vi "ring_buoy_ring.vi"(8 "error in (no error)":errorcluster, 11 "Image":T1) -> (0 "error out":errorcluster, 2 "circular particles":dbl[][](array[numeric]), 3 "Image Dst Out":T1)   [LabVIEW 2009]
uses:
  <vilib>/vision/Image Controls.llb/IMAQ Image.ctl
  <vilib>/vision/NI_Vision_Development_Module.lvlib
panel:
  out "size(s)":i32[](array[numeric])
  out "Particle Measurements (Pixels)":dbl[][](array[numeric]) format="%.2f"
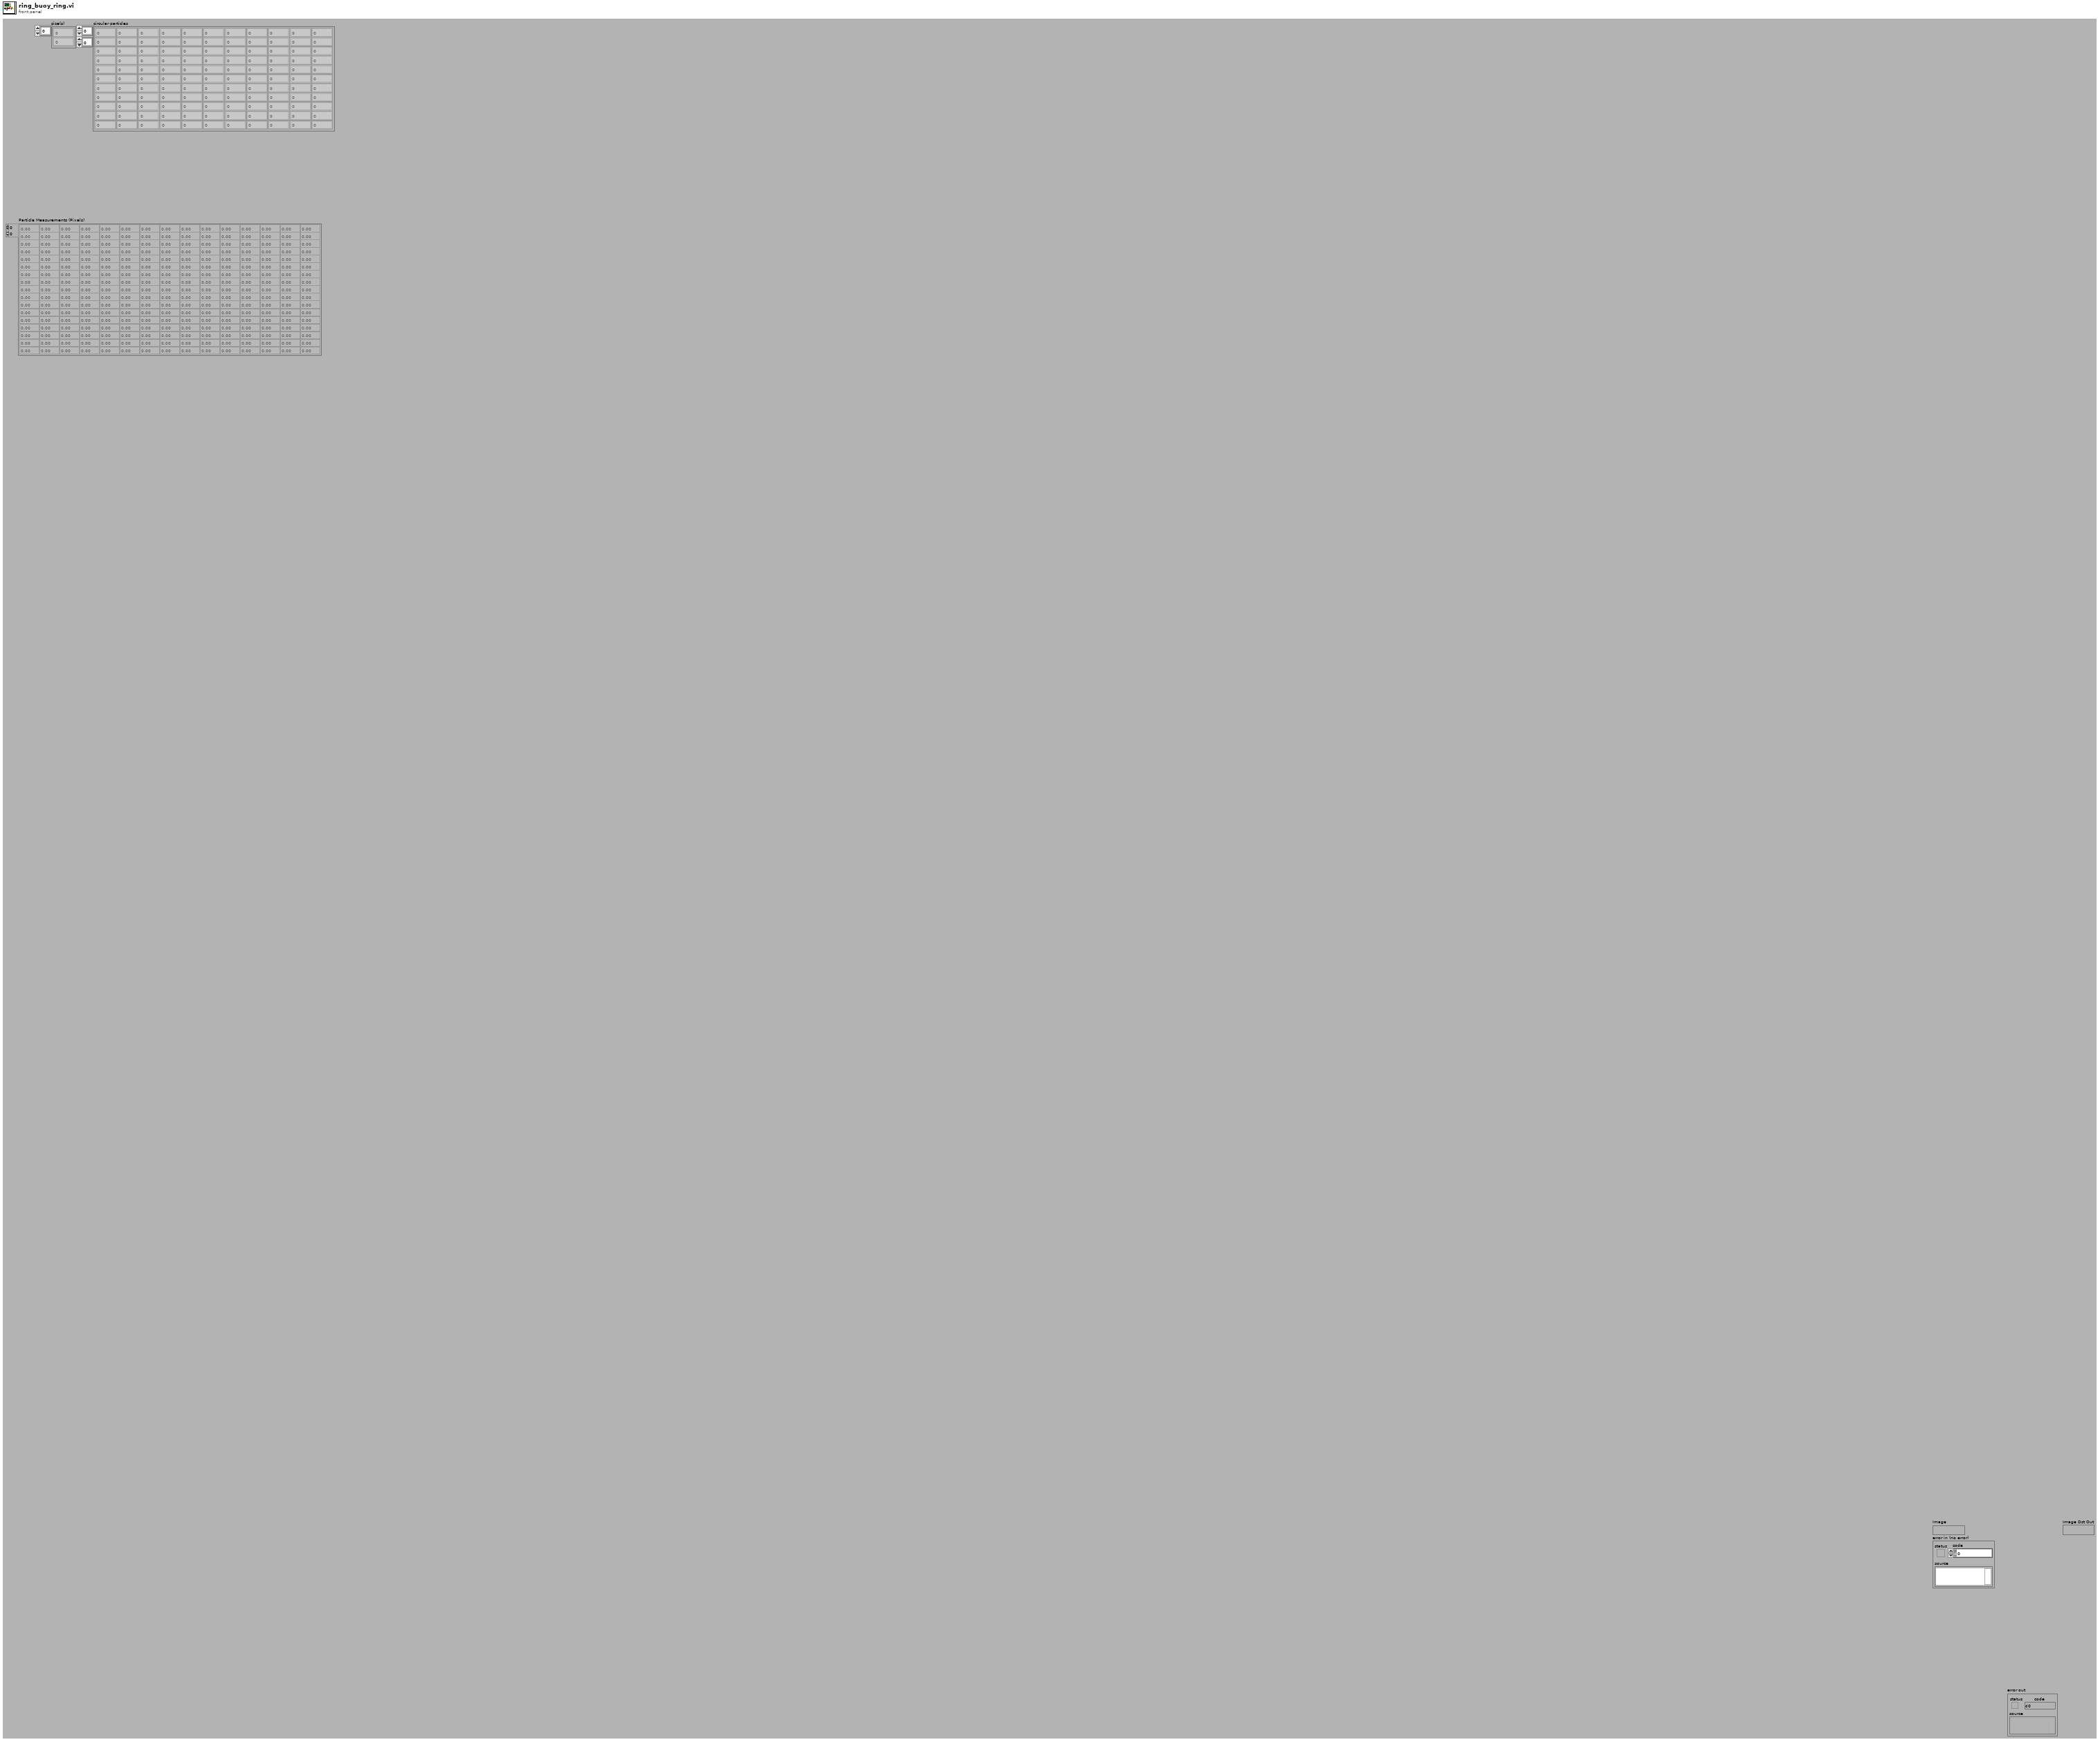
[diagram p1: front panel]
types:
  T1 = typedef "IMAQ Image.ctl" = refnum<image>
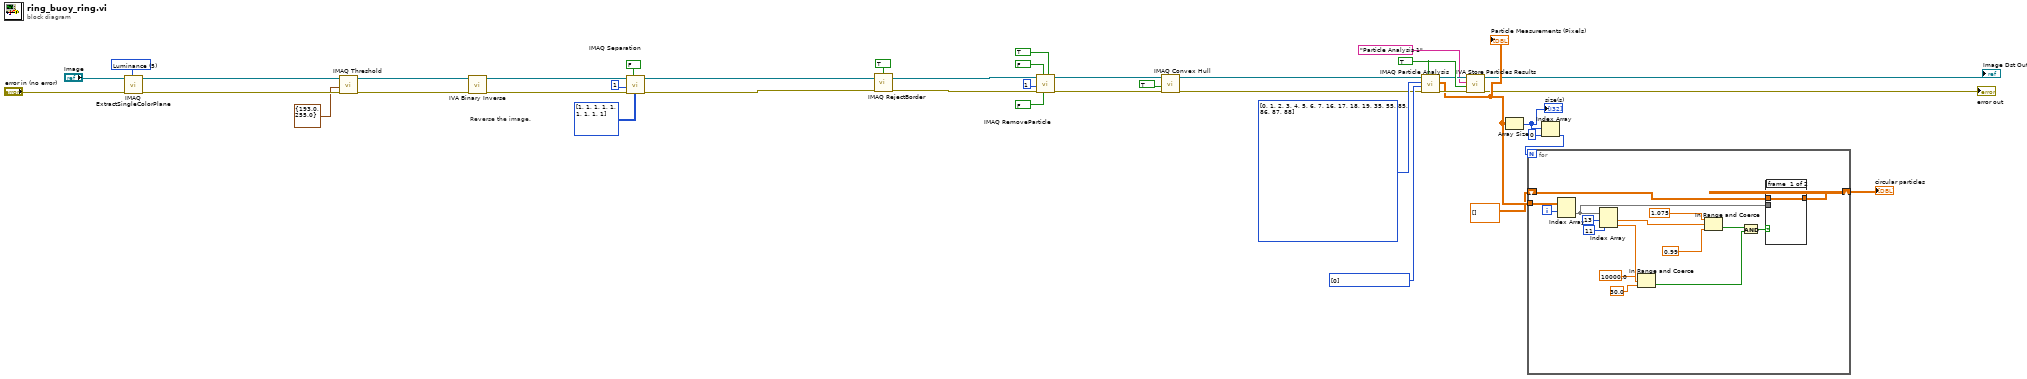
[diagram p0: block diagram]
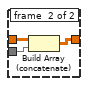
[diagram p2: hidden frame]
diagram:
  w16 = i32[] [0] items=["Center of Mass X", "Center of Mass Y", "First Pixel X", "First Pixel Y", "Bounding Rect Left", "Bounding Rect Top", "Bounding Rect Right", "Bounding Rect Bottom", "Max Feret Diameter Start X", "Max Feret Diameter Start Y", "Max Feret Diameter End X", "Max Feret Diameter End Y", "Max Horiz. Segment Length Left", "Max Horiz. Segment Length Right", "Max Horiz. Segment Length Row", "-", "Bounding Rect Width", "Bounding Rect Height", "Bounding Rect Diagonal", "Perimeter", "Convex Hull Perimeter", "Holes' Perimeter", "Max Feret Diameter", "Equivalent Ellipse Major Axis", "Equivalent Ellipse Minor Axis", "Equivalent Ellipse Minor Axis (Feret)", "Equivalent Rect Long Side", "Equivalent Rect Short Side", "Equivalent Rect Diagonal", "Equivalent Rect Short Side (Feret)", "Average Horiz. Segment Length", "Average Vert. Segment Length", "Hydraulic Radius", "Waddel Disk Diameter", "-", "Area", "Holes' Area", "Particle & Holes' Area", "Convex Hull Area", "Image Area", "-", "Number of Holes", "Number of Horiz. Segments", "Number of Vert. Segments", "-", "Orientation", "Max Feret Diameter Orientation", "-", "% Area/Image Area", "% Area/(Particle & Holes' Area)", "Ratio of Equivalent Ellipse Axes", "Ratio of Equivalent Rect Sides", "-", "Elongation Factor", "Compactness Factor", "Heywood Circularity Factor", "Type Factor", "-", "Sum X", "Sum Y", "Sum XX", "Sum XY", "Sum YY", "Sum XXX", "Sum XXY", "Sum XYY", "Sum YYY", "-", "Moment of Inertia XX", "Moment of Inertia XY", "Moment of Inertia YY", "Moment of Inertia XXX", "Moment of Inertia XXY", "Moment of Inertia XYY", "Moment of Inertia YYY", "Norm. Moment of Inertia XX", "Norm. Moment of Inertia XY", "Norm. Moment of Inertia YY", "Norm. Moment of Inertia XXX", "Norm. Moment of Inertia XXY", "Norm. Moment of Inertia XYY", "Norm. Moment of Inertia YYY", "Hu Moment 1", "Hu Moment 2", "Hu Moment 3", "Hu Moment 4", "Hu Moment 5", "Hu Moment 6", "Hu Moment 7"] ("Real-World Measurements")
  w11 = i32[] [0, 1, 2, 3, 4, 5, 6, 7, 16, 17, 18, 19, 35, 55, 85, 86, 87, 88] items=["Center of Mass X", "Center of Mass Y", "First Pixel X", "First Pixel Y", "Bounding Rect Left", "Bounding Rect Top", "Bounding Rect Right", "Bounding Rect Bottom", "Max Feret Diameter Start X", "Max Feret Diameter Start Y", "Max Feret Diameter End X", "Max Feret Diameter End Y", "Max Horiz. Segment Length Left", "Max Horiz. Segment Length Right", "Max Horiz. Segment Length Row", "-", "Bounding Rect Width", "Bounding Rect Height", "Bounding Rect Diagonal", "Perimeter", "Convex Hull Perimeter", "Holes' Perimeter", "Max Feret Diameter", "Equivalent Ellipse Major Axis", "Equivalent Ellipse Minor Axis", "Equivalent Ellipse Minor Axis (Feret)", "Equivalent Rect Long Side", "Equivalent Rect Short Side", "Equivalent Rect Diagonal", "Equivalent Rect Short Side (Feret)", "Average Horiz. Segment Length", "Average Vert. Segment Length", "Hydraulic Radius", "Waddel Disk Diameter", "-", "Area", "Holes' Area", "Particle & Holes' Area", "Convex Hull Area", "Image Area", "-", "Number of Holes", "Number of Horiz. Segments", "Number of Vert. Segments", "-", "Orientation", "Max Feret Diameter Orientation", "-", "% Area/Image Area", "% Area/(Particle & Holes' Area)", "Ratio of Equivalent Ellipse Axes", "Ratio of Equivalent Rect Sides", "-", "Elongation Factor", "Compactness Factor", "Heywood Circularity Factor", "Type Factor", "-", "Sum X", "Sum Y", "Sum XX", "Sum XY", "Sum YY", "Sum XXX", "Sum XXY", "Sum XYY", "Sum YYY", "-", "Moment of Inertia XX", "Moment of Inertia XY", "Moment of Inertia YY", "Moment of Inertia XXX", "Moment of Inertia XXY", "Moment of Inertia XYY", "Moment of Inertia YYY", "Norm. Moment of Inertia XX", "Norm. Moment of Inertia XY", "Norm. Moment of Inertia YY", "Norm. Moment of Inertia XXX", "Norm. Moment of Inertia XXY", "Norm. Moment of Inertia XYY", "Norm. Moment of Inertia YYY", "Hu Moment 1", "Hu Moment 2", "Hu Moment 3", "Hu Moment 4", "Hu Moment 5", "Hu Moment 6", "Hu Moment 7"] ("Pixel Measurements")
  w15 = TRUE ("Connectivity 4/8 (8)")
  w41 = 5 items=["Red", "Green", "Blue", "Hue", "Saturation", "Luminance", "Value", "Intensity"] ("Color Plane")
  # "Reverse the image."
  n1 = call "IMAQ ExtractSingleColorPlane"("Color Plane"=w41, "error in (no error)"="error in (no error)", "Image Src"="Image") -> ("error out"=w40:errorcluster, "Image Dst Out"=w38:T1)  [unwired: 1 in, 6 out]
  n2 = call "IMAQ Threshold"("error in (no error)"=w40, "Range"=cluster{"Lower value":sgl, "Upper value":sgl} {"Lower value"=193.0, "Upper value"=255.0}, "Image Src"=w38) -> ("error out"=w37:errorcluster, "Image Dst Out"=w36:T1)  [unwired: 3 in, 4 out]
  n3 = call <vilib>:"IVA Binary Inverse.vi"("error in (no error)"=w37, "Image In"=w36) -> ("error out"=w35:errorcluster, "Image Out"=w31:T1)  [unwired: 8 out]
  n4 = call "IMAQ Separation"("Structuring Element"=i32[][] [[1, 1, 1], [1, 1, 1], [1, 1, 1]], "Square/Hexa (Square)"=FALSE, "error in (no error)"=w35, "Nb of Erosion"=1, "Image Src"=w31) -> ("error out"=w19:errorcluster, "Image Dst Out"=w20:T1)  [unwired: 1 in, 4 out]
  n5 = call "IMAQ RejectBorder"("error in (no error)"=w19, "Image Src"=w20, "Connectivity 4/8 (8)"=TRUE) -> ("error out"=w29:errorcluster, "Image Dst Out"=w24:T1)  [unwired: 1 in, 2 out]
  n6 = call "IMAQ RemoveParticle"("Connectivity 4/8 (8)"=TRUE, "Low Pass/High Pass (Low)"=FALSE, "Square/Hexa (Square)"=FALSE, "error in (no error)"=w29, "Number of Erosion"=1, "Image Src"=w24) -> ("error out"=w17:errorcluster, "Image Dst Out"=w18:T1)  [unwired: 1 in, 3 out]
  n7 = call "IMAQ Convex Hull"("error in (no error)"=w17, "Connectivity 4/8 (8)"=TRUE, "Image Src"=w18) -> ("error out"=w3:errorcluster, "Image Dst Out"=w4:T1)  [unwired: 1 in, 6 out]
  n8 = call "IMAQ Particle Analysis"("Connectivity 4/8 (8)"=w15, "error in (no error)"=w3, "Real-World Measurements"=w16, "Pixel Measurements"=w11, "Image"=w4) -> ("error out"=w12:errorcluster, "Particle Measurements (Pixels)"=w10:dbl[][], "Image Out (duplicate)"=w14:T1)  [unwired: 4 out]
  "Particle Measurements (Pixels)" <- w10
  n9 = call <vilib>:"IVA Store Particles Results.vi"("error in (no error)"=w12, "Connectivity 4/8 (8)"=w15, "Step Name"="Particle Analysis 1", "Image in"=w14) -> ("error out"=→"error out":errorcluster, "Image dup"=→"Image Dst Out":T1)  [unwired: 6 out]
  n10 = Array Size(array=w10) -> (size(s)=w9:i32[])
  "size(s)" <- w9
  n11 = Index Array(array=w9, index=0) -> (element=w7:i32)
  n12 = for {
    N: w7 -> [_]
    tunnel: w10 -> [w57]
    shift-right: [w52] -> w5
    shift-left: dbl[][] [] ("Particle Measurements (Pixels)") -> [w55]
    i -> [w56]
    n13 = Index Array(array=w57, index (row)=w56) -> (element=w53:dbl[])  [unwired: 1 in]
    n14 = Index Array(array=w53, index #1=13 ("index"), index #2=11 ("index")) -> (element #1=w51:dbl, element #2=w47:dbl)
    n15 = In Range and Coerce(upper limit=10000.0, x=w47, lower limit=30.0) -> (In Range?=w42:bool)  [unwired: 1 out]
    n16 = In Range and Coerce(upper limit=1.075 ("max circularity"), x=w51, lower limit=0.99 ("y")) -> (In Range?=w43:bool)  [unwired: 1 out]
    n17 = And(x=w43, y=w42) -> (x .and. y?=w44:bool)
    n18 = case shown="True" w44 {
      tunnel: w55 -> [w58 w61]
      tunnel: w53 -> [_ w60]
      tunnel: [w58 w59] -> w52
      frame #0 {
      }
      frame #1 {
        n19 = Build Array (concatenate)(w61, w60) -> (w59:dbl[][])
      }
    }
  }
  "circular particles" <- w5
